vi "Configuration UI.vi"(8 "error in":errorcluster, 11 "Message ni":T1={"This VI Ref"=refnum, "Test VI"=refnum, "Q Ref"=refnum, "UE"=refnum, "Data"=variant, "Timeout"=-1, "Path List[]"=[], "Status"="", "Counter"=0, "Config"={"Source Path"=path "", "Dest Path"=path "", "Log Path"=path "", "Move?"=FALSE, "Log?"=FALSE, "Scanners"=[], "Excude Folders"=[], "Jpg?"=FALSE, "Default path"=path "", "Extended?"=FALSE, "Mode"=enum."Move", "Temp"=FALSE}, "Total"=0, "Config Path"=path "", "exif info"={"Make"="Canon\u0000", "Model"="Canon PowerShot A495\u0000", "Orientation"=0, "Date"=timestamp(0 s since 1904-01-01), "Width"=0, "Height"=0, "Square?"=FALSE, "File Name"="Canon\u0000", "Extension"="Canon\u0000", "Valid?"=FALSE, "Path"=path "", "size"=0, "No Ext?"=FALSE, "prefix?"=FALSE, "String"="", "Name Type"=enum."Event Sufix"}, "app operation"=enum."Start", "Log Ref"=refnum, "Start Time"=0.0, "Pause Time"=0.0, "Argument?"=FALSE, "Argument path"=path "", "Identical"=FALSE, "File.lvclass"=refnum}) -> (0 "error out":errorcluster, 3 "Message out":T1={"This VI Ref"=refnum, "Test VI"=refnum, "Q Ref"=refnum, "UE"=refnum, "Data"=variant, "Timeout"=-1, "Path List[]"=[], "Status"="", "Counter"=0, "Config"={"Source Path"=path "", "Dest Path"=path "", "Log Path"=path "", "Move?"=FALSE, "Log?"=FALSE, "Scanners"=[], "Excude Folders"=[], "Jpg?"=FALSE, "Default path"=path "", "Extended?"=FALSE, "Mode"=enum."Move", "Temp"=FALSE}, "Total"=0, "Config Path"=path "", "exif info"={"Make"="Canon\u0000", "Model"="Canon PowerShot A495\u0000", "Orientation"=0, "Date"=timestamp(0 s since 1904-01-01), "Width"=0, "Height"=0, "Square?"=FALSE, "File Name"="Canon\u0000", "Extension"="Canon\u0000", "Valid?"=FALSE, "Path"=path "", "size"=0, "No Ext?"=FALSE, "prefix?"=FALSE, "String"="", "Name Type"=enum."Event Sufix"}, "app operation"=enum."Start", "Log Ref"=refnum, "Start Time"=0.0, "Pause Time"=0.0, "Argument?"=FALSE, "Argument path"=path "", "Identical"=FALSE, "File.lvclass"=refnum})   [LabVIEW 2023, in "User Interface.lvlib"]
uses:
  User Interface.lvlib
  Controls/main consumer cluster.ctl
  File Classes/File/File.lvclass
  Controls/configuration cluster.ctl
  File Classes/Controls/exif data cluster.ctl
  File Classes/Controls/rename type enum.ctl
  Controls/app operation state enum.ctl
  File Classes/File Classes.lvlib
panel:
  in  "Cancel":bool
  in  "Shell":bool
  in  "Extended?":bool
  in  "Default Path (%userprofile%\\Pictures)":path
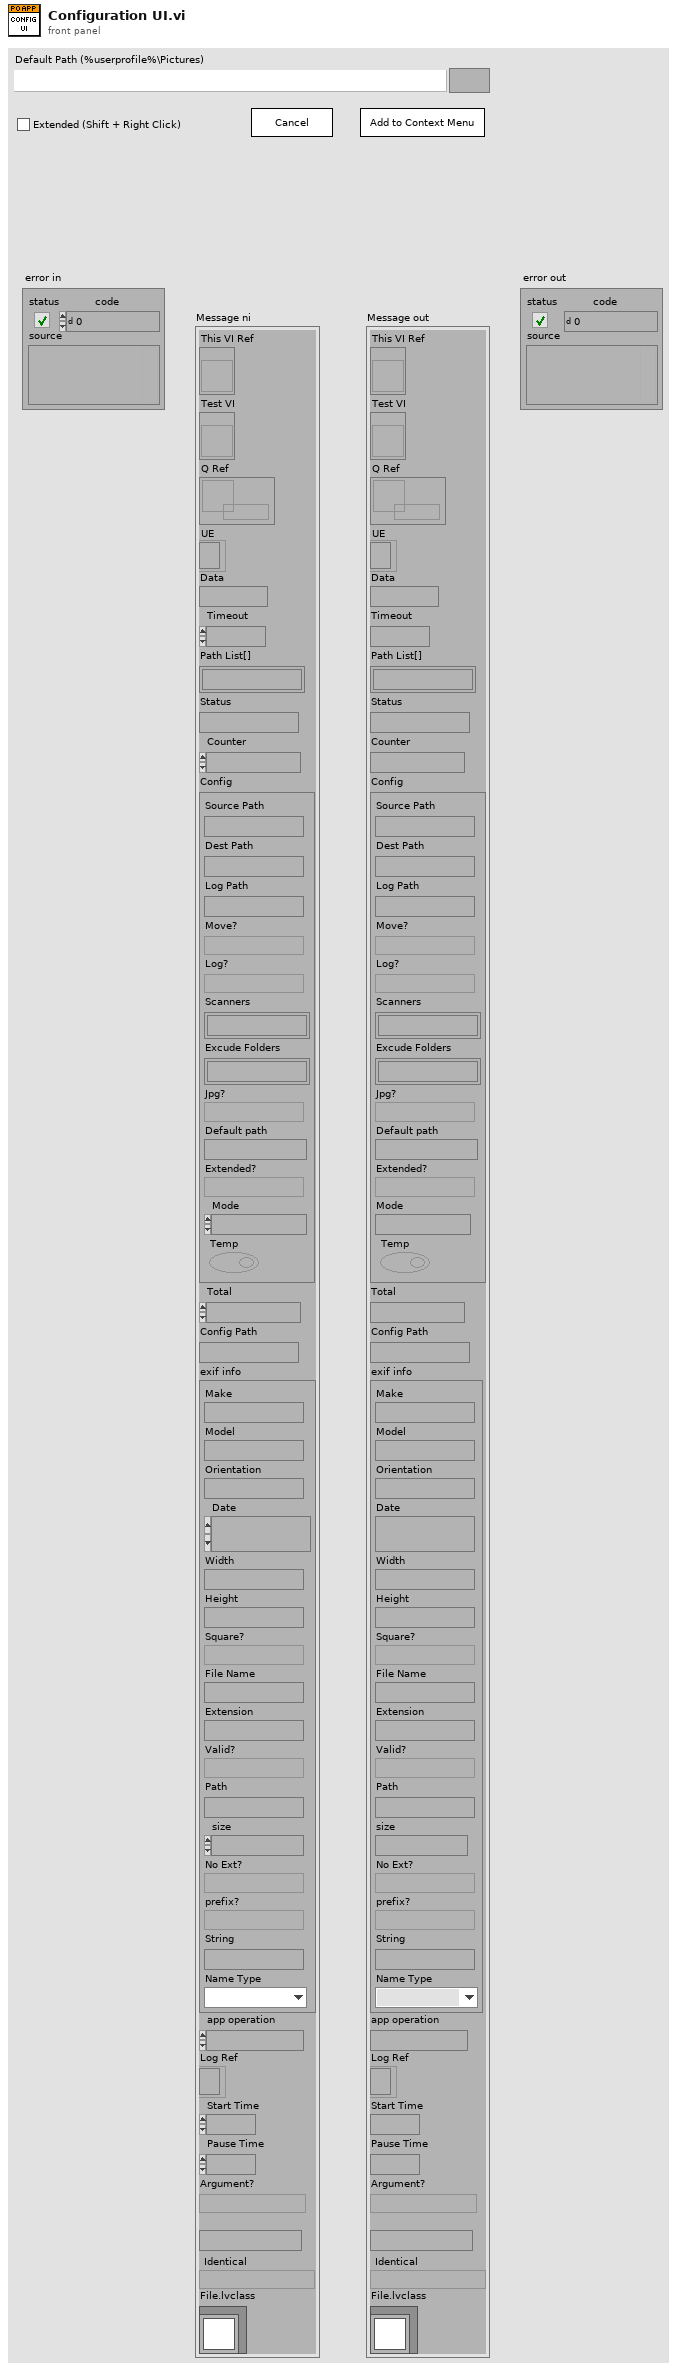
[diagram p1: front panel]
types:
  T1 = typedef "User Interface.lvlib/main consumer cluster.ctl" = cluster{"This VI Ref":refnum<vi>, "Test VI":refnum<vi>, "Q Ref":refnum<queue>, "UE":refnum<event-registration>, "Data":variant, "Timeout":i32, "Path List[]":path[], "Status":string, "Counter":i32, "Config":T2, "Total":i32, "Config Path":path, "exif info":T3, "app operation":T5, "Log Ref":refnum<file>, "Start Time":dbl, "Pause Time":dbl, "Argument?":bool, "Argument path":path, "Identical":bool, "File.lvclass":refnum<class "File.lvclass">}
  T2 = typedef "User Interface.lvlib/configuration cluster.ctl" = cluster{"Source Path":path, "Dest Path":path, "Log Path":path, "Move?":bool, "Log?":bool, "Scanners":string[], "Excude Folders":string[], "Jpg?":bool, "Default path":path, "Extended?":bool, "Mode":enum16{"Copy (Default)", "Move", "Rename"}, "Temp":bool}
  T3 = typedef "File Classes.lvlib/exif data cluster.ctl" = cluster{"Make":string, "Model":string, "Orientation":u16, "Date":timestamp, "Width":u16, "Height":u16, "Square?":bool, "File Name":string, "Extension":string, "Valid?":bool, "Path":path, "size":i64, "No Ext?":bool, "prefix?":bool, "String":string, "Name Type":T4}
  T4 = typedef "File Classes.lvlib/rename type enum.ctl" = enum16{"Date & Time (Default)", "Model Sufix", "Event Sufix", "Model & Event Sufix"}
  T5 = typedef "User Interface.lvlib/app operation state enum.ctl" = enum16{"Start", "Stop", "Pause", "Resume"}
  T6 = typedef "User Interface.lvlib/registry settings cluster.ctl" = cluster{"App Key":string, "Context Label":string, "Command":string, "Position":enum16{"Top", "Middle", "Bottom"}, "Extended?":bool, "Location":enum16{"File - Root", "Ext - Root", "Directory - Root", "File - Classes", "Ext - Classes", "Folder - Classes", "Dir Bak Gnd - Root"}, "Icon path":string, "Ext (No Dot)":string}
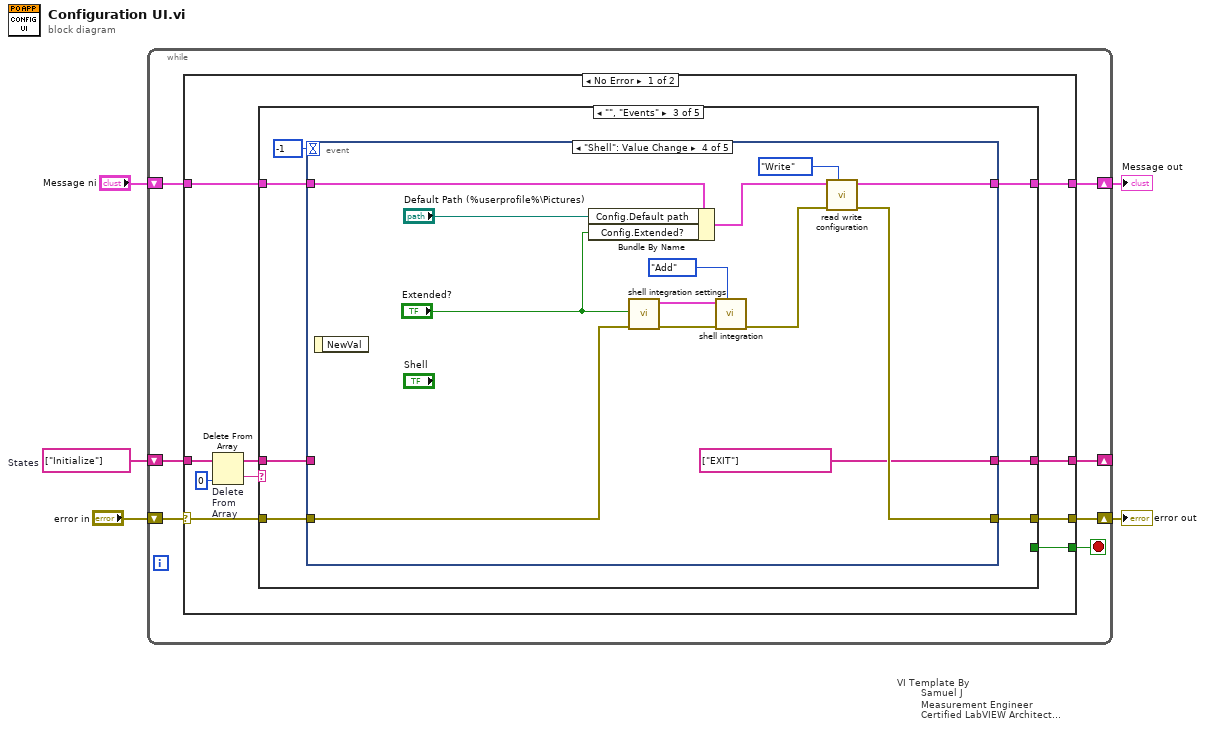
[diagram p0: block diagram]
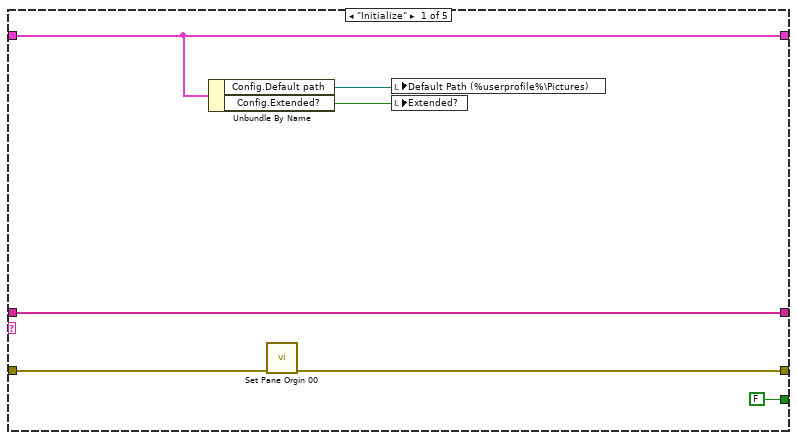
[diagram p2: hidden frame]
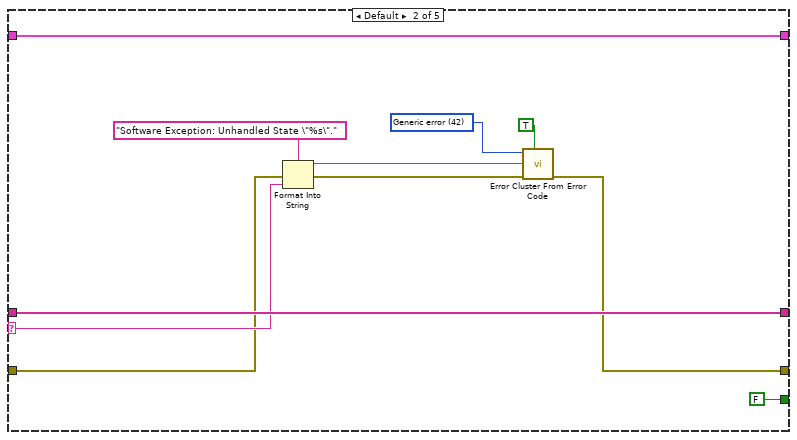
[diagram p3: hidden frame]
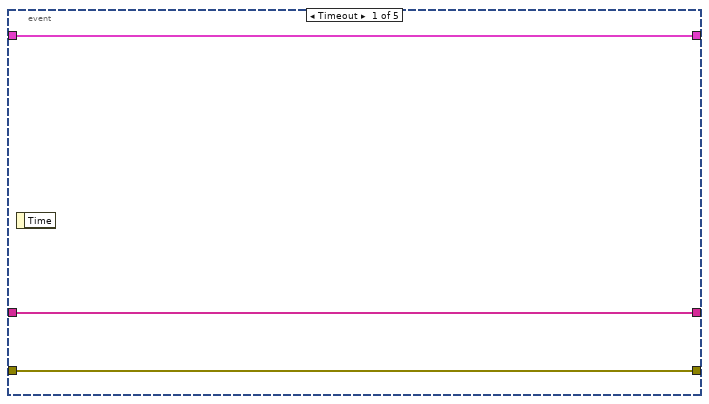
[diagram p4: hidden frame]
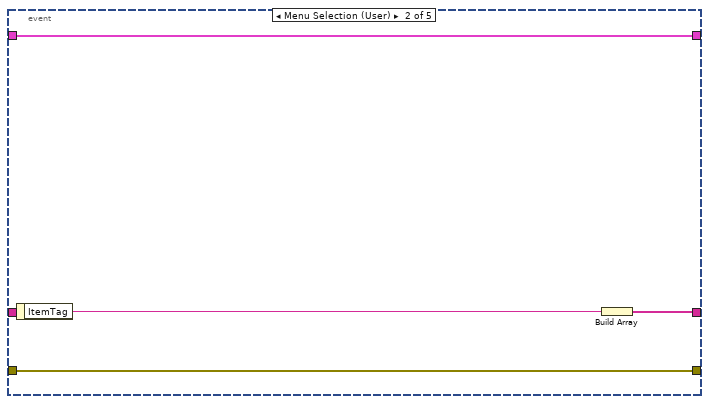
[diagram p5: hidden frame]
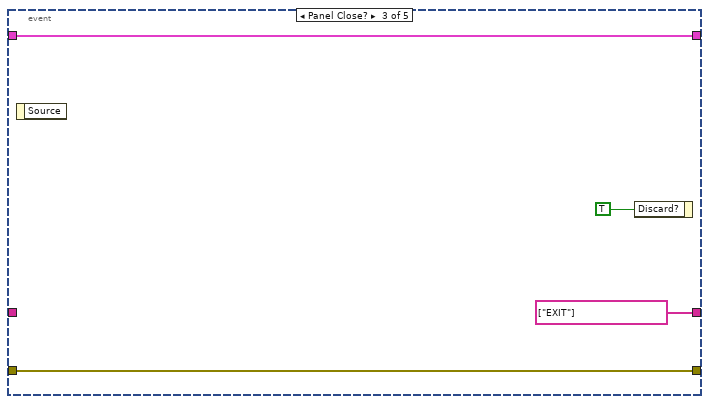
[diagram p6: hidden frame]
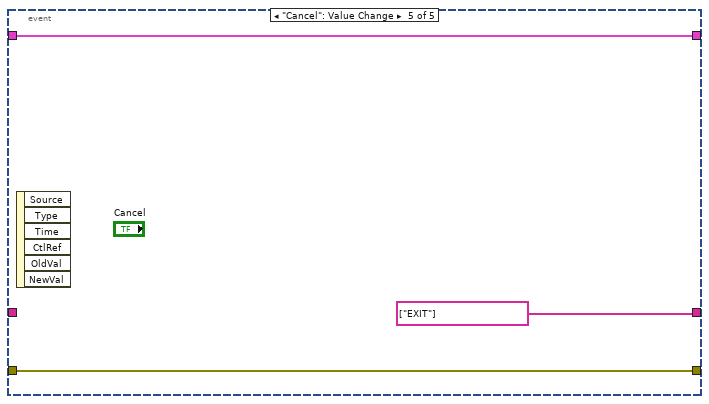
[diagram p7: hidden frame]
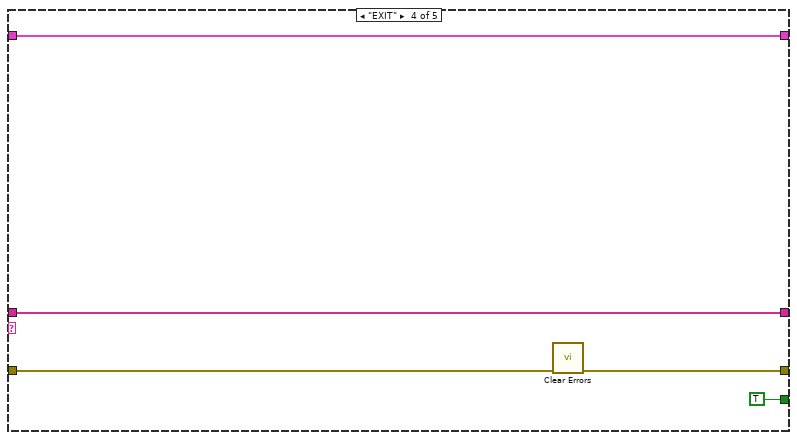
[diagram p8: hidden frame]
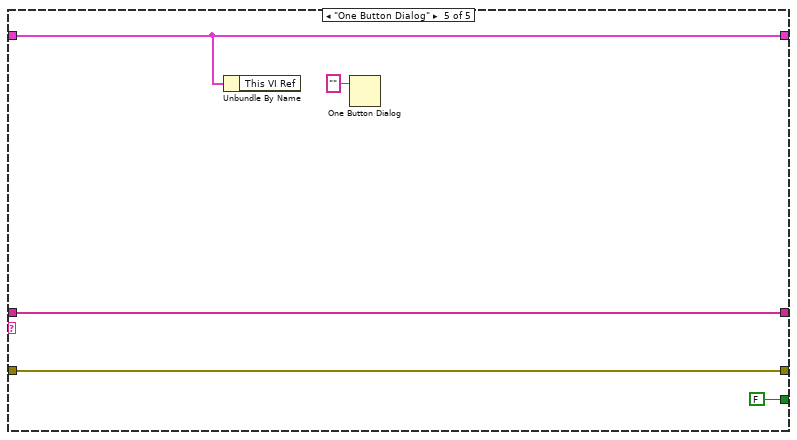
[diagram p9: hidden frame]
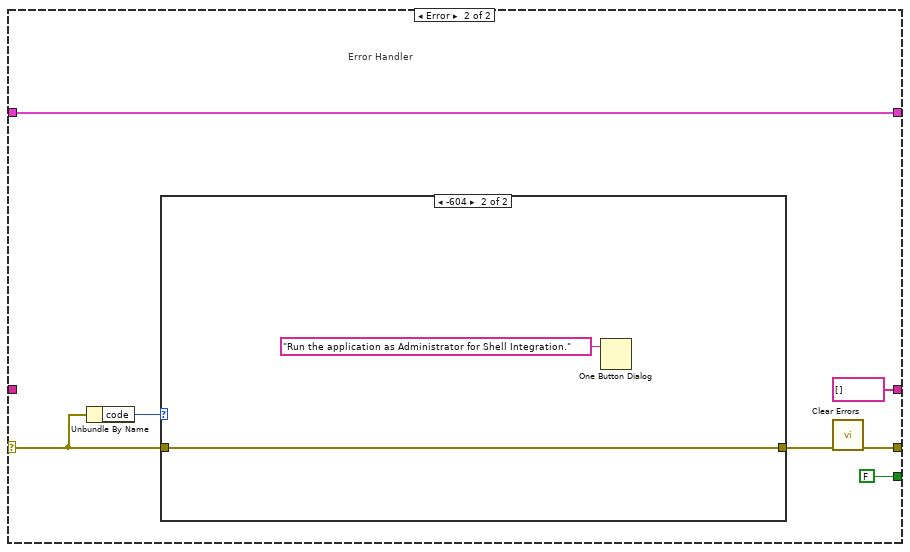
[diagram p10: hidden frame]
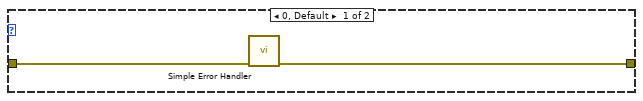
[diagram p11: hidden frame]
diagram:
  w5 = string[] ["Initialize"]  # States
  n1 = while "VI Template By\n        Samuel J\n        Measurement Engineer\n        Certified LabVIEW Architect\n        Vestas Technology R&D Chennai" {
    shift-right: [w8] -> _
    shift-left: w5 -> [w12]
    shift-right: [w9] -> w1
    shift-left: "error in" -> [w11]
    shift-right: [w7] -> w2
    shift-left: "Message ni" -> [w10]
    stop <- w6 stop-if-true
    n2 = case shown="No Error" w11 {
      selector: w11 -> [w17 w89]
      tunnel: w12 -> [w21 _]
      tunnel: w10 -> [w18 w91]
      tunnel: [w16 w87] -> w9
      tunnel: [w15 string[] [] ("States")] -> w8
      tunnel: [w14 w91] -> w7
      tunnel: [w13 FALSE ("Exit")] -> w6
      frame No Error {
        n3 = Delete From Array "Delete\nFrom\nArray"(array=w21, index=0) -> (deleted portion=w20:string, array with subset deleted=w19:string[])  [unwired: 1 in]
        n4 = case shown="\"\", \"Events\"" w20 {
          selector: w20 -> [_ w32 _ _ _]
          tunnel: w19 -> [w29 w40 w42 w79 w83]
          tunnel: w18 -> [w25 w39 w47 w78 w82]
          tunnel: w17 -> [w27 w31 w46 w75 w84]
          tunnel: [w26 w30 w44 w76 w84] -> w16
          tunnel: [w29 w40 w43 w79 w83] -> w15
          tunnel: [w25 w39 w45 w78 w82] -> w14
          tunnel: [FALSE ("Exit") FALSE ("Exit") _ TRUE ("Exit") FALSE ("Exit")] -> w13
          frame "Initialize" {
            n5 = Unbundle By Name(w25) -> ("Config.Default path"=w24:path, "Config.Extended?"=w23:bool)
            n6 = call <userlib>:"Set Pane Orgin 00.vi"("error in"=w27) -> ("error out"=w26:errorcluster)  [unwired: 10 in]
            n7 = local write "Default Path (%userprofile%\\Pictures)"(w24) -> ()
            n8 = local write "Extended?"(w23) -> ()
          }
          frame Default {
            w34 = 42 items=["No error", "Argument error", "Memory is full", "Out of zone", "End of file", "File already open", "Generic file I/O error", "File not found", "File permission error", "Disk is full", "Duplicate path", "Too many files open", "System feature not enabled", "Resource file not found", "Cannot add resource", "Resource not found", "Image not found", "Image memory error", "Pen does not exist", "Config type invalid", "Config token not found", "Config parse error", "Config memory error", "Bad external code format", "Bad external code offset", "External code not present", "Null window", "Destroy window error", "Null menu", "Print aborted", "Bad print record", "Print driver error", "Windows error during printing", "Memory error during printing", "Print dialog error", "Generic print error", "Invalid device refnum", "Device not found", "Device parameter error", "Device unit error", "Cannot open device", "Device call aborted", "Generic error", "Cancelled by user", "Object ID too low", "Object ID too high", "Object not in heap", "Unknown heap", "Unknown object (invalid DefProc)", "Unknown object (DefProc not in table)", "Message out of range", "Invalid (null) method", "Unknown message", "Manager call not supported", "Bad address", "Network operation in progress", "Network operation timed out", "Connection is busy", "Network attribute not supported", "Network error", "Address in use", "System out of memory", "Connection aborted", "Connection refused", "Not connected", "Already connected", "Connection closed", "Initialization error (interapplication manager)", "Bad occurrence", "Wait on unbound occurrence handler", "Occurrence queue overflow", "Datalog type conflict", "Unused", "Unrecognized type (interapplication manager)", "Memory corrupt", "Failed to make temporary DLL", "Old CIN version", "Drag socket not found", "Failed to load drop-object", "Failed to register OLE object", "Failed to release OLE object", "Format specifier type mismatch", "Unknown format specifier", "Too few format specifiers", "Too many format specifiers", "Scan failed", "Newer CIN version", "Error converting to variant", "Runtime menu error", "Password tampered", "Variant attribute not found", "Incompatible variant data type", "Event data is not available", "Event Store is not present", "Occurrence is not found", "Event Queue is not created", "Event info is not available", "Refnum passed is NULL", "Error retrieving Class GUID", "Error retrieving CoClass GUID", "Error retrieving TypeLib GUID.", "Bad built application magic bytes.", "Specific driver is different from the specific driver associated with the Logical Name.", "There is no session opened to the class driver.", "Max Error", "MAX - Error with config objects", "MAX - Error loading configuration", "MAX - Group not supported"]
            n9 = Format Into String(format string="Software Exception: Unhandled State \"%s\"." ("message"), error in=w31, w32) -> (resulting string=w35:string, error out=w36:errorcluster)  [unwired: 1 in]
            n10 = call <vilib>:"Error Cluster From Error Code.vi"("show call chain? (False)"=TRUE, "error in (no error)"=w36, "error message (\"\")"=w35, "error code (0)"=w34) -> ("error out"=w30:errorcluster)  [unwired: 5 out]
          }
          frame "", "Events" {
            n11 = event shown="[3] \"Shell\": Value Change" {
              selector: _ -> [_ _ _ _ _]
              dyn-events: _ -> [_ _ _ _ _]
              timeout: -1 -> [_ _ _ _ _]
              tunnel: w47 -> [w50 w54 w57 w63 w74]
              tunnel: w46 -> [w49 w51 w56 w65 w73]
              tunnel: [w50 w54 w57 w68 w74] -> w45
              tunnel: [w49 w51 w56 w64 w73] -> w44
              tunnel: [w48 w52 string[] ["EXIT"] ("States") string[] ["EXIT"] ("States") string[] ["EXIT"] ("States")] -> w43
              tunnel: w42 -> [w48 _ _ _ _]
              event Timeout {
                n12 = event-data() -> ()  [unwired: 2 out]
              }
              event Menu Selection (User) {
                n13 = event-data() -> ("ItemTag"=w53:string)  [unwired: 1 out]
                n14 = Build Array(w53) -> (w52:string[])
              }
              event Panel Close? {
                n15 = event-data() -> ()  [unwired: 2 out]
                n16 = event-data("Discard?"=TRUE) -> ()  [unwired: 1 in, 1 out]
              }
              event "Shell": Value Change {
                n17 = event-data() -> ()  [unwired: 2 out]
                n18 = Bundle By Name(cluster=w63, "Config.Default path"="Default Path (%userprofile%\\Pictures)", "Config.Extended?"="Extended?") -> (w62:T1)
                n19 = call "shell integration settings.vi"("error in"=w65, "Extended?"="Extended?") -> ("error out"=w71:errorcluster, "cluster out"=w70:T6)  [unwired: 8 in]
                n20 = call "shell integration.vi"("Command"=enum16{"Add", "Remove"}."Add", "error in"=w71, "Cluster"=w70) -> ("error out"=w66:errorcluster)  [unwired: 7 in, 1 out]
                n21 = call "read write configuration.vi"("Enum"=enum16{"Read", "Write"}."Write", "error in"=w66, "Consumer Cluster in"=w62) -> ("error out"=w64:errorcluster, "cluster out"=w68:T1)  [unwired: 7 in]
              }
              event "Cancel": Value Change {
                n22 = event-data() -> ()  [unwired: 7 out]
              }
            }
          }
          frame "EXIT" {
            n23 = call <vilib>:"Clear Errors.vi"("error in (no error)"=w75) -> ("error out"=w76:errorcluster)  [unwired: 5 in, 1 out]
          }
          frame "One Button Dialog" {
            n24 = Unbundle By Name(w82) -> ()  [unwired: 1 out]
            n25 = One Button Dialog(message="") -> ()  [unwired: 2 out]
          }
        }
      }
      frame Error {
        # "Error Handler"
        n26 = Unbundle By Name(w89) -> ("code"=w90:i32)
        n27 = case shown="-604" w90 {
          tunnel: w89 -> [w93 w95]
          tunnel: [w92 w95] -> w88
          frame 0, Default {
            n28 = call <vilib>:"Simple Error Handler.vi"("error in (no error)"=w93) -> ("error out"=w92:errorcluster)  [unwired: 1 in, 7 out]
          }
          frame -604 {
            n29 = One Button Dialog(message="Run the application as Administrator for Shell Integration.") -> ()  [unwired: 2 out]
          }
        }
        n30 = call <vilib>:"Clear Errors.vi"("error in (no error)"=w88) -> ("error out"=w87:errorcluster)  [unwired: 1 in, 5 out]
      }
    }
  }
  "Message out" <- w2
  "error out" <- w1
